vi "Init.vi"(3 "Container State":T3, 4 "Previous State":variant, 5 "Previous Version":T2) -> (2 "Current State":T1={"Update"=FALSE, "Show advanced"=FALSE, "Fs (Hz)"=100000.0, "Show persist"=FALSE})   [LabVIEW 2020, in "Stimulus Channel (Full).xctl"]
uses:
  Stimulus Channel (Full).xctl
  State.ctl
  <vilib>/_xctls/Container State.ctl
  <vilib>/_xctls/Version.ctl
  State V1.ctl
  <vilib>/_xctls/XControlSupport.lvlib
panel:
  in  "Default Indicator State":T1={"Update"=FALSE, "Show advanced"=FALSE, "Fs (Hz)"=100000.0, "Show persist"=FALSE}
  in  "Default Control State":T1={"Update"=FALSE, "Show advanced"=FALSE, "Fs (Hz)"=100000.0, "Show persist"=FALSE}
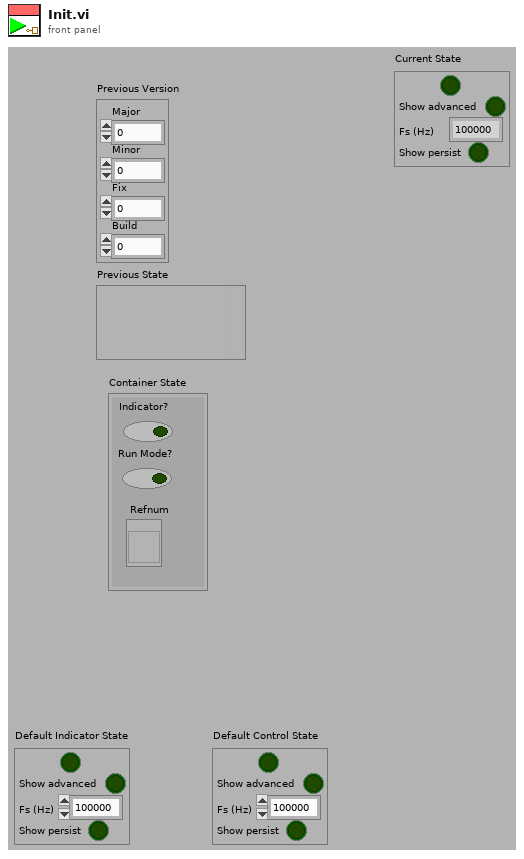
[diagram p1: front panel]
types:
  T1 = typedef "Stimulus Channel (Full).xctl/State.ctl" = cluster{"Update":bool, "Show advanced":bool, "Fs (Hz)":dbl, "Show persist":bool}
  T2 = typedef "XControlSupport.lvlib/Version.ctl" = cluster{"Major":u16, "Minor":u16, "Fix":u16, "Build":u16}
  T3 = typedef "XControlSupport.lvlib/Container State.ctl" = cluster{"Indicator?":bool, "Run Mode?":bool, " Refnum":refnum<vi>}
  T4 = typedef "Stimulus Channel (Full).xctl/State V1.ctl" = cluster{"Update":bool, "Show advanced":bool, "Fs (Hz)":dbl}
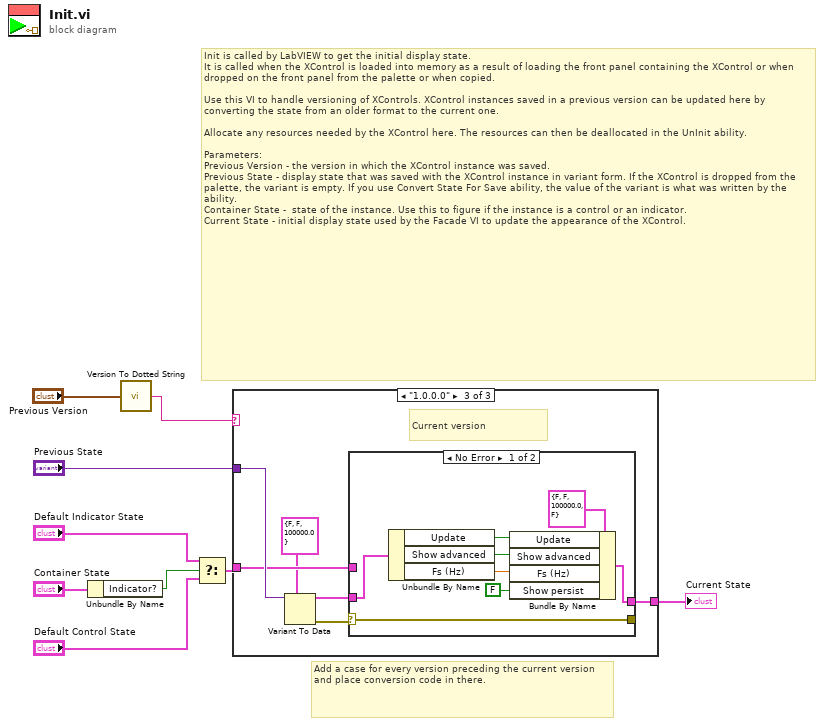
[diagram p0: block diagram]
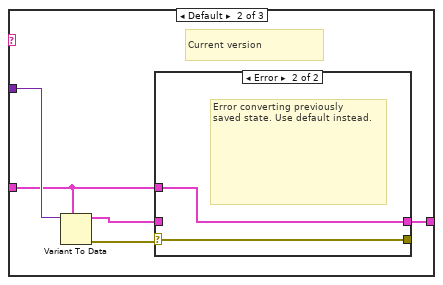
[diagram p3: hidden frame]
diagram:
  # "Add a case for every version preceding the current version and place conversion code in there."
  # "Init is called by LabVIEW to get the initial display state.\nIt is called when the XControl is loaded into memory as a result of loading the front panel containing the XControl or when dropped on the front panel from the palette or when copied.\n\nUse this VI to handle versioning of XControls. XControl instances saved in a previous version can be updated here by converting the state from an older format to the current one.\n\nAllocate any resources needed by the XControl here. The resources can then be deallocated in the UnInit ability.\n\nParameters:\nPrevious Version - the version in which the XControl instance was saved.\nPrevious State - display state that was saved with the XControl instance in variant form. If the XControl is dropped from the palette, the variant is empty. If you use Convert State For Save ability, the value of the variant is what was written by the ability. \nContainer State -  state of the instance. Use this to figure if the instance is a control or an indicator.\nCurrent State - initial display state used by the Facade VI to update the appearance of the XControl."
  n1 = Unbundle By Name("Container State") -> ("Indicator?"=w4:bool)
  n2 = call <vilib>:"Version To Dotted String.vi"("Version"="Previous Version") -> ("String Version"=w1:string)
  n3 = Select(t="Default Indicator State", s=w4, f="Default Control State") -> (s? t:f=w3:T1)
  n4 = case shown="\"1.0.0.0\"" w1 {
    tunnel: "Previous State" -> [_ w15 w25]
    tunnel: [w10 w11 w21] -> w8
    tunnel: w3 -> [w10 w12 w22]
    frame "0.0.0.0" {
      # "Just created, use default state"
    }
    frame Default {
      # "Current version"
      n5 = Variant To Data(type=w12, Variant=w15) -> (data=w13:T1, error out=w14:errorcluster)  [unwired: 1 in]
      n6 = case shown="Error" w14 {
        selector: w14 -> [w17 w18]
        tunnel: w13 -> [w16 _]
        tunnel: [w16 w19] -> w11
        tunnel: w12 -> [_ w19]
        tunnel: [w17 w18] -> _
        frame No Error {
        }
        frame Error {
          # "Error converting previously \nsaved state. Use default instead."
        }
      }
    }
    frame "1.0.0.0" {
      # "Current version"
      n7 = Variant To Data(type=T4 {"Update"=FALSE, "Show advanced"=FALSE, "Fs (Hz)"=100000.0} ("State"), Variant=w25) -> (data=w23:T4, error out=w24:errorcluster)  [unwired: 1 in]
      n8 = case shown="No Error" w24 {
        selector: w24 -> [w33 w34]
        tunnel: w23 -> [w32 _]
        tunnel: [w28 w35] -> w21
        tunnel: w22 -> [_ w35]
        tunnel: [w33 w34] -> _
        frame No Error {
          n9 = Unbundle By Name(w32) -> ("Update"=w30:bool, "Show advanced"=w29:bool, "Fs (Hz)"=w27:dbl)
          n10 = Bundle By Name(cluster=T1 {"Update"=FALSE, "Show advanced"=FALSE, "Fs (Hz)"=100000.0, "Show persist"=FALSE} ("State"), "Update"=w30, "Show advanced"=w29, "Fs (Hz)"=w27, "Show persist"=FALSE) -> (w28:T1)
        }
        frame Error {
          # "Error converting previously \nsaved state. Use default instead."
        }
      }
    }
  }
  "Current State" <- w8
